vi "加标回收量程配置界面.vi"(3 "量程选择簇":T1={"氨氮推荐量程"=enum."AUTO", "总氮推荐量程"=enum."AUTO", "总磷推荐量程"=enum."AUTO", "CODMn推荐量程"=enum."H", "CODCr推荐量程"=enum."H"}, 11 "倒计时":u16) -> (2 "布尔":bool=TRUE)   [LabVIEW 2016]
uses:
  <vilib>/Utility/miscctls.llb/LVPointTypeDef.ctl
  <vilib>/Utility/config.llb/NI_LVConfig.lvlib
panel:
  in  "确认":bool
  in  "返回":bool
  in  "详情":bool
  out "CODCr 2":dbl
  out "CODMn 2":dbl
  out "总磷 2":dbl
  out "总氮 2":dbl
  out "氨氮 2":dbl
  in  "取消":bool
  out "CODCr":dbl
  out "CODMn":dbl
  out "总磷":dbl
  out "总氮":dbl
  out "氨氮":dbl
  out "CODCr下限":dbl
  out "CODCr上限":dbl
  out "CODMn下限":dbl
  out "CODMn上限":dbl
  out "总磷下限":dbl
  out "总磷上限":dbl
  out "总氮下限":dbl
  out "总氮上限":dbl
  out "氨氮下限":dbl
  out "氨氮上限":dbl
  # "加标回收量程选择"
  # "最近一组水样测试结果"
  # "加标后的理论浓度"
  # "氨氮低量程范围"
  # "~"
  # "总氮低量程范围"
  # "~"
  # "总磷低量程范围"
  # "~"
  # "~"
  # "CODMn低量程范围"
  # "~"
  # "CODCr低量程范围"
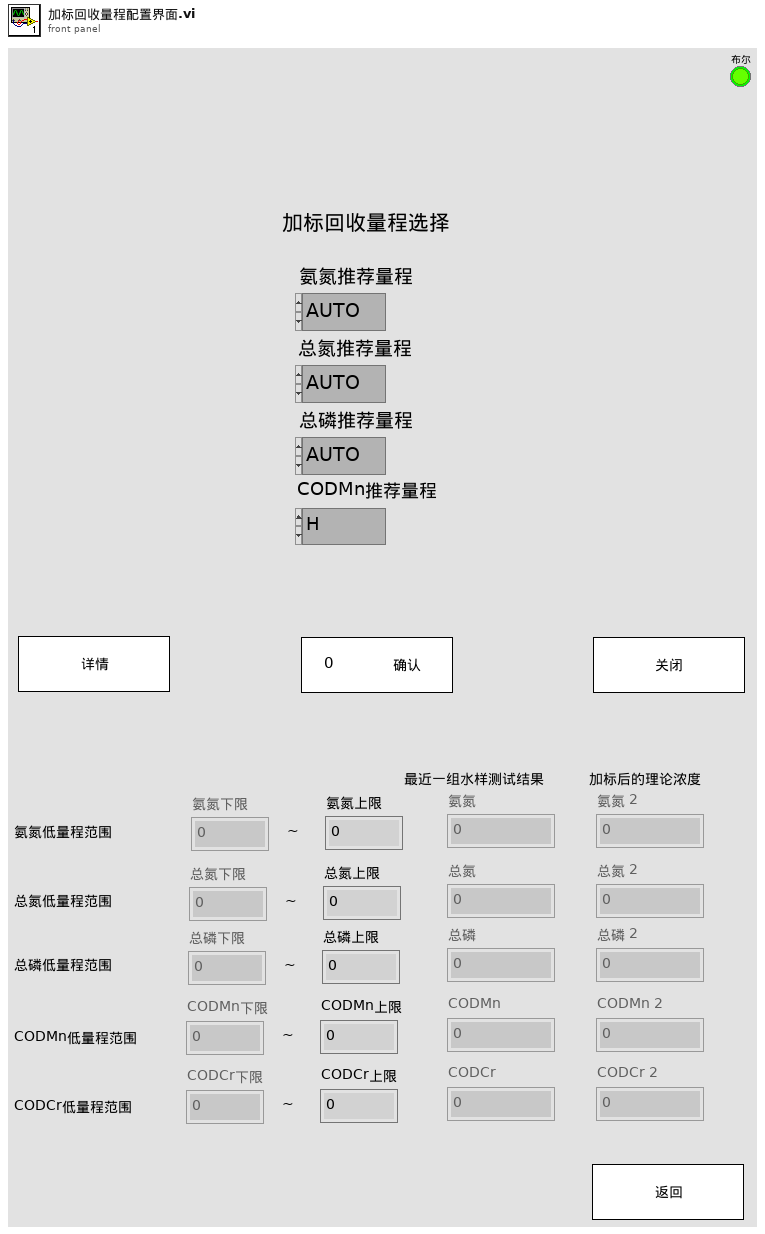
[diagram p1: front panel]
types:
  T1 = cluster{"氨氮推荐量程":enum32{"H", "L", "AUTO"}, "总氮推荐量程":enum32{"H", "L", "AUTO"}, "总磷推荐量程":enum32{"H", "L", "AUTO"}, "CODMn推荐量程":enum32{"H", "L", "AUTO"}, "CODCr推荐量程":enum32{"H", "L", "AUTO"}}
  T2 = cluster{"量程":dbl, "检出限":dbl, "加标前水样浓度":dbl, "加标后水样浓度":dbl, "加标水杯定容体积":dbl, "加标母液浓度":dbl, "加标体积":dbl, "加标回收率":dbl}
  T3 = typedef "NI_LVConfig.lvlib/Config Data RefNum.ctl" = refnum<k1>
  T4 = typedef "LVPointTypeDef.ctl" = cluster{"Horizontal":i16, "Vertical":i16}
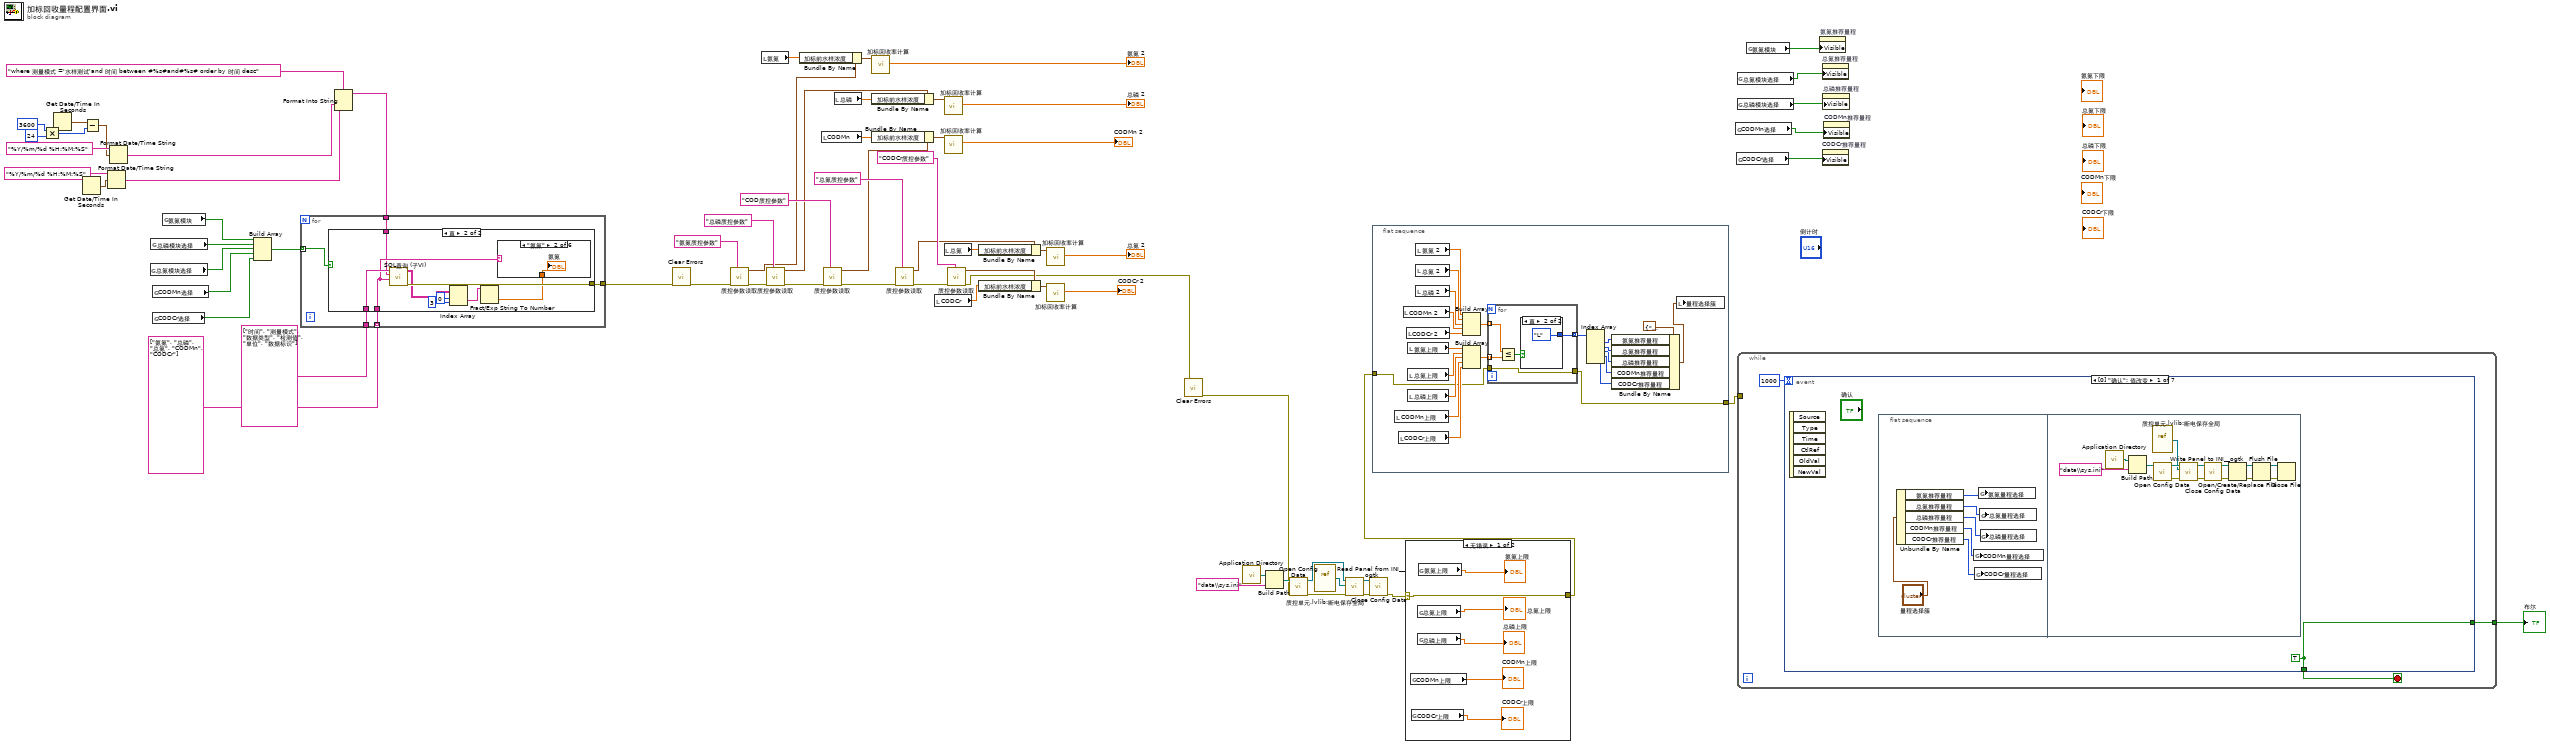
[diagram p0: block diagram]
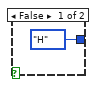
[diagram p2: hidden frame]
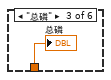
[diagram p5: hidden frame]
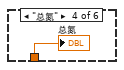
[diagram p6: hidden frame]
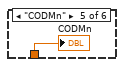
[diagram p7: hidden frame]
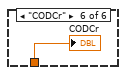
[diagram p8: hidden frame]
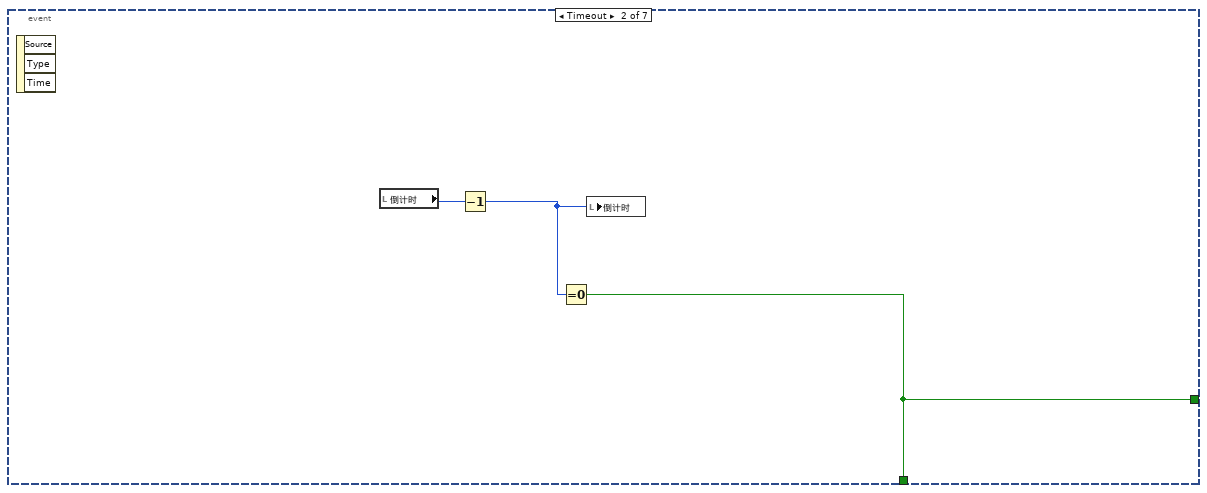
[diagram p10: hidden frame]
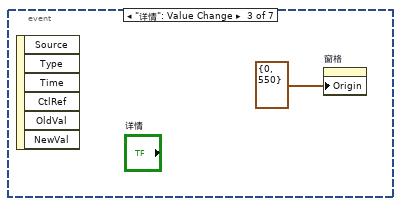
[diagram p11: hidden frame]
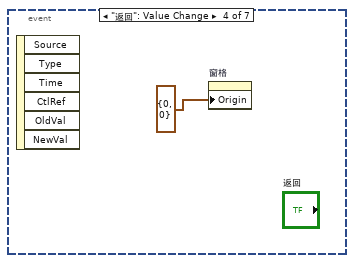
[diagram p12: hidden frame]
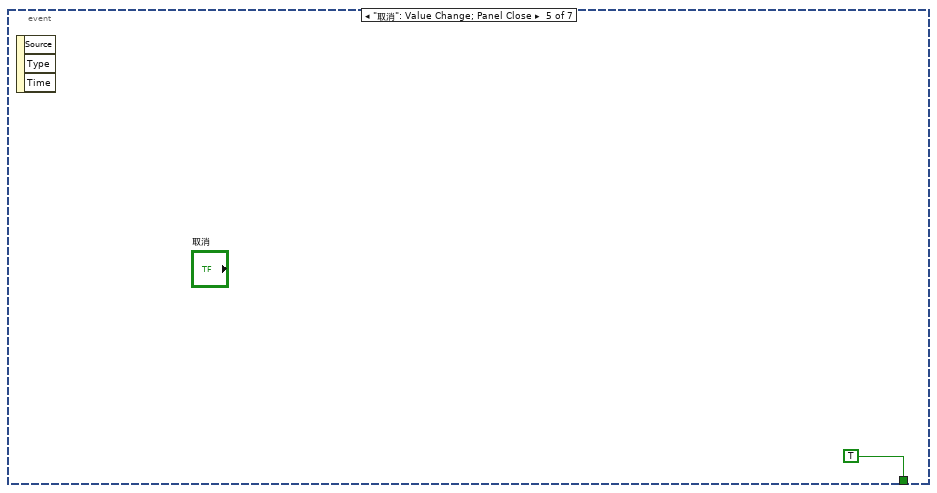
[diagram p13: hidden frame]
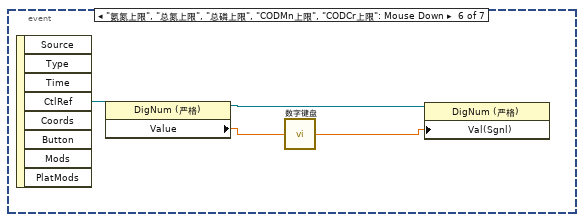
[diagram p14: hidden frame]
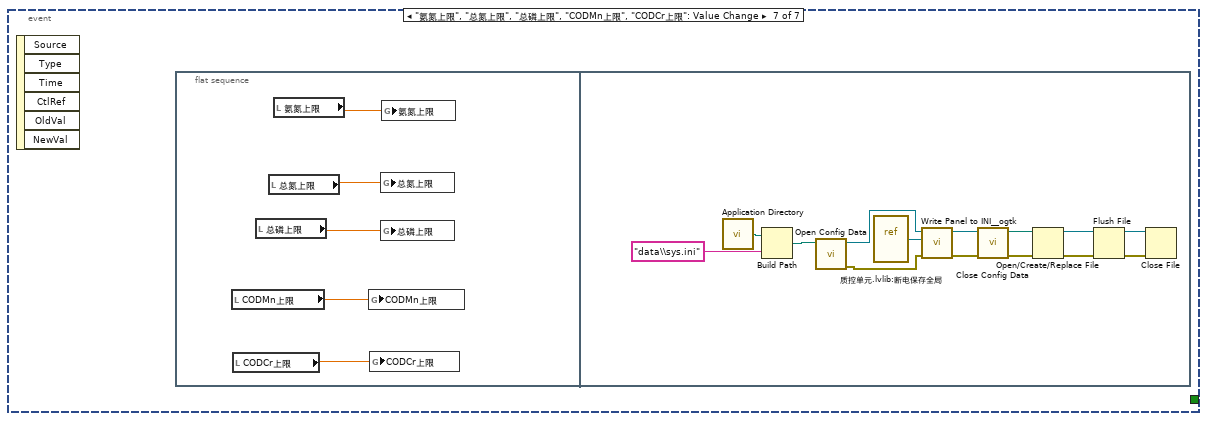
[diagram p15: hidden frame]
diagram:
  n1 = Multiply(x=3600, y=24) -> (x*y=w46:i32)
  n2 = Get Date/Time In Seconds() -> (seconds since 1Jan1904=w50:timestamp)
  n3 = Get Date/Time In Seconds() -> (seconds since 1Jan1904=w53:timestamp)
  n4 = Subtract(x=w50, y=w46) -> (x-y=w49:timestamp)
  n5 = Format Date/Time String(time format string (%c)="%Y/%m/%d %H:%M:%S" ("时间格式字符串(%c)"), seconds (now)=w53) -> (date/time string=w43:string)  [unwired: 1 in]
  n6 = Format Date/Time String(time format string (%c)="%Y/%m/%d %H:%M:%S" ("时间格式字符串(%c)"), seconds (now)=w49) -> (date/time string=w44:string)  [unwired: 1 in]
  n7 = global read "断电保存全局.vi" "总氮模块选择"() -> (w59:bool)
  n8 = global read "断电保存全局.vi" "总磷模块选择"() -> (w60:bool)
  n9 = global read "断电保存全局.vi" "CODMn选择"() -> (w58:bool)
  n10 = global read "断电保存全局.vi" "CODCr选择"() -> (w57:bool)
  n11 = global read "断电保存全局.vi" "氨氮模块"() -> (w61:bool)
  n12 = Build Array(w61, w60, w59, w58, w57) -> (w56:bool[])
  n13 = Format Into String(format string="where 测量模式 ='水样测试'and 时间 between #%s#and#%s# order by 时间 desc", w44, w43) -> (resulting string=w42:string)  [unwired: 2 in, 1 out]
  n14 = for {
    tunnel: w56 -> [w75] mode=indexing
    tunnel: string[] ["氨氮", "总磷", "总氮", "CODMn", "CODCr"] -> [w74] mode=indexing
    tunnel: string[] ["时间", "测量模式", "数据类型", "检测值", "单位", "数据标识"] ("columns") -> [w73]
    tunnel: [w72] -> w32
    tunnel: w42 -> [w71]
    n15 = case shown="真" w75 {
      tunnel: w74 -> [_ w82]
      tunnel: w73 -> [_ w84]
      tunnel: [_ w83] -> w72
      tunnel: w71 -> [_ w81]
      frame False {
      }
      frame True {
        n16 = call "SQL查询 (子VI).vi"("table输入"=w82, "condition"=w81, "columns"=w84) -> ("错误输出"=w83:errorcluster, "data"=w77:string[][])  [unwired: 7 in]
        n17 = Index Array(array=w77, index (row)=0 ("索引 (行)"), index (col)=3 ("禁用的索引 (列)")) -> (element=w80:string)
        n18 = Fract/Exp String To Number(string=w80) -> (number=w76:dbl)  [unwired: 3 in, 1 out]
        n19 = case shown="\"氨氮\"" w82 {
          tunnel: w76 -> [_ w85 w86 w87 w88 w89]
          frame "假", Default {
          }
          frame "氨氮" {
            "氨氮" <- w85
          }
          frame "总磷" {
            "总磷" <- w86
          }
          frame "总氮" {
            "总氮" <- w87
          }
          frame "CODMn" {
            "CODMn" <- w88
          }
          frame "CODCr" {
            "CODCr" <- w89
          }
        }
      }
    }
  }
  n20 = call <vilib>:"Clear Errors.vi"("error in (no error)"=w32) -> ("error out"=w31:errorcluster)  [unwired: 5 in, 1 out]
  n21 = call "质控参数读取.vi"("section"="氨氮质控参数", "error in (no error)"=w31) -> ("error out"=w39:errorcluster, "参数"=w30:T2)  [unwired: 8 in]
  n22 = local read "氨氮"() -> (w29:dbl)
  n23 = call "质控参数读取.vi"("section"="总磷质控参数", "error in (no error)"=w39) -> ("error out"=w37:errorcluster, "参数"=w24:T2)  [unwired: 8 in]
  n24 = Bundle By Name(cluster=w30, "加标前水样浓度"=w29) -> (w28:T2)
  n25 = local read "CODMn"() -> (w21:dbl)
  n26 = call "质控参数读取.vi"("section"="COD质控参数", "error in (no error)"=w37) -> ("error out"=w35:errorcluster, "参数"=w20:T2)  [unwired: 8 in]
  n27 = local read "总磷"() -> (w25:dbl)
  n28 = call "加标回收率计算.vi"("参数"=w28) -> ("加标后理论浓度"=→"氨氮 2":dbl)  [unwired: 9 in, 1 out]
  n29 = Bundle By Name(cluster=w24, "加标前水样浓度"=w25) -> (w26:T2)
  n30 = Bundle By Name(cluster=w20, "加标前水样浓度"=w21) -> (w22:T2)
  n31 = call "质控参数读取.vi"("section"="总氮质控参数", "error in (no error)"=w35) -> ("error out"=w33:errorcluster, "参数"=w16:T2)  [unwired: 8 in]
  n32 = local read "CODCr"() -> (w13:dbl)
  n33 = call "加标回收率计算.vi"("参数"=w26) -> ("加标后理论浓度"=→"总磷 2":dbl)  [unwired: 9 in, 1 out]
  n34 = call "加标回收率计算.vi"("参数"=w22) -> ("加标后理论浓度"=→"CODMn 2":dbl)  [unwired: 9 in, 1 out]
  n35 = local read "总氮"() -> (w18:dbl)
  n36 = call "质控参数读取.vi"("section"="CODCr质控参数", "error in (no error)"=w33) -> ("error out"=w10:errorcluster, "参数"=w12:T2)  [unwired: 8 in]
  n37 = Bundle By Name(cluster=w16, "加标前水样浓度"=w18) -> (w17:T2)
  n38 = Bundle By Name(cluster=w12, "加标前水样浓度"=w13) -> (w14:T2)
  n39 = call "加标回收率计算.vi"("参数"=w17) -> ("加标后理论浓度"=→"总氮 2":dbl)  [unwired: 9 in, 1 out]
  n40 = call "加标回收率计算.vi"("参数"=w14) -> ("加标后理论浓度"=→"CODCr 2":dbl)  [unwired: 9 in, 1 out]
  n41 = call <vilib>:"Clear Errors.vi"("error in (no error)"=w10) -> ("error out"=w9:errorcluster)  [unwired: 5 in, 1 out]
  n42 = call <vilib>:"Application Directory.vi"() -> ("Application Directory"=w70:path)
  n43 = Build Path(base path=w70, name or relative path="data\\sys.ini" ("名称或相对路径")) -> (appended path=w68:path)
  n44 = call <vilib>:"Open Config Data.vi"("error in (no error)"=w9, "configuration file path"=w68) -> ("error out"=w64:errorcluster, "refnum"=w67:T3)  [unwired: 7 in, 1 out]
  n45 = vi-ref "质控单元.lvlib:断电保存全局.vi"() -> (w66:refnum<vi>)
  n46 = call <userlib>:"Read Panel from INI__ogtk.vi"("error in (no error)"=w64, "VI ref"=w66, "refnum"=w67) -> ("error out"=w63:errorcluster, "refnum out"=w65:T3)  [unwired: 7 in]
  n47 = call <vilib>:"Close Config Data.vi"("error in (no error)"=w63, "refnum"=w65) -> ("error out"=w62:errorcluster)  [unwired: 8 in, 1 out]
  n48 = flat-sequence {
    tunnel: w8 -> [w98]
    tunnel: [w97] -> w7
    frame #0 {
      n49 = local read "CODMn上限"() -> (w102:dbl)
      n50 = local read "CODCr上限"() -> (w101:dbl)
      n51 = local read "CODMn 2"() -> (w107:dbl)
      n52 = local read "CODCr 2"() -> (w108:dbl)
      n53 = local read "氨氮上限"() -> (w105:dbl)
      n54 = local read "总氮上限"() -> (w104:dbl)
      n55 = local read "总磷上限"() -> (w103:dbl)
      n56 = local read "氨氮 2"() -> (w111:dbl)
      n57 = local read "总氮 2"() -> (w110:dbl)
      n58 = local read "总磷 2"() -> (w109:dbl)
      n59 = Build Array(w111, w110, w109, w107, w108) -> (w106:dbl[])
      n60 = Build Array(w105, w104, w103, w102, w101) -> (w100:dbl[])
      n61 = for {
        tunnel: w106 -> [w116] mode=indexing
        tunnel: w100 -> [w115] mode=indexing
        tunnel: [w114] -> w99 mode=indexing
        tunnel: w98 -> [w112]
        tunnel: [w112] -> w97
        n62 = Less Or Equal?(x=w116, y=w115) -> (x <= y?=w113:bool)
        n63 = case shown="真" w113 {
          tunnel: [enum32{"H", "L", "AUTO"}."H" ("氨氮推荐量程") enum32{"H", "L", "AUTO"}."L" ("氨氮推荐量程")] -> w114
          frame False {
          }
          frame True {
          }
        }
      }
      n64 = Index Array(array=w99) -> (element #1=w95:enum32{"H", "L", "AUTO"}, element #2=w94:enum32{"H", "L", "AUTO"}, element #3=w93:enum32{"H", "L", "AUTO"}, element #4=w92:enum32{"H", "L", "AUTO"}, element #5=w91:enum32{"H", "L", "AUTO"})  [unwired: 5 in]
      n65 = Bundle By Name(cluster=T1 {"氨氮推荐量程"=enum."H", "总氮推荐量程"=enum."H", "总磷推荐量程"=enum."H", "CODMn推荐量程"=enum."H", "CODCr推荐量程"=enum."H"} ("量程选择簇"), "氨氮推荐量程"=w95, "总氮推荐量程"=w94, "总磷推荐量程"=w93, "CODMn推荐量程"=w92, "CODCr推荐量程"=w91) -> (w90:T1)
      n66 = local write "量程选择簇"(w90) -> ()
    }
  }
  n67 = case shown="无错误" w62 {
    selector: w62 -> [w119 w125]
    tunnel: [w119 w125] -> w8
    frame No Error {
      n68 = global read "断电保存全局.vi" "CODMn上限"() -> (→"CODMn上限":dbl)
      n69 = global read "断电保存全局.vi" "CODCr上限"() -> (→"CODCr上限":dbl)
      n70 = global read "断电保存全局.vi" "总氮上限"() -> (→"总氮上限":dbl)
      n71 = global read "断电保存全局.vi" "总磷上限"() -> (→"总磷上限":dbl)
      n72 = global read "断电保存全局.vi" "氨氮上限"() -> (→"氨氮上限":dbl)
    }
    frame Error {
    }
  }
  n73 = global read "断电保存全局.vi" "CODMn选择"() -> (w3:bool)
  n74 = global read "断电保存全局.vi" "CODCr选择"() -> (w4:bool)
  n75 = global read "断电保存全局.vi" "总氮模块选择"() -> (w1:bool)
  n76 = global read "断电保存全局.vi" "总磷模块选择"() -> (w2:bool)
  n77 = while {
    tunnel: w7 -> [_]
    tunnel: [w127] -> w6
    stop <- w128 stop-if-true
    n78 = event shown="[0] \"确认\": 值改变" {
      selector: _ -> [_ _ _ _ _ _ _]
      dyn-events: _ -> [_ _ _ _ _ _ _]
      timeout: 1000 -> [_ _ _ _ _ _ _]
      tunnel: [w129 w151 _ _ TRUE _ _] -> w128
      tunnel: [w129 w151 _ _ _ _ _] -> w127
      event "确认": Value Change {
        w129 = TRUE
        n79 = event-data() -> ()  [unwired: 1 in, 6 out]
        n80 = flat-sequence {
          frame #0 {
            n81 = Unbundle By Name("量程选择簇") -> ("氨氮推荐量程"=w135:enum32{"H", "L", "AUTO"}, "总氮推荐量程"=w134:enum32{"H", "L", "AUTO"}, "总磷推荐量程"=w133:enum32{"H", "L", "AUTO"}, "CODMn推荐量程"=w132:enum32{"H", "L", "AUTO"}, "CODCr推荐量程"=w131:enum32{"H", "L", "AUTO"})
            n82 = global write "断电保存全局.vi" "CODMn量程选择"(w132) -> ()
            n83 = global write "断电保存全局.vi" "CODCr量程选择"(w131) -> ()
            n84 = global write "断电保存全局.vi" "氨氮量程选择"(w135) -> ()
            n85 = global write "断电保存全局.vi" "总氮量程选择"(w134) -> ()
            n86 = global write "断电保存全局.vi" "总磷量程选择"(w133) -> ()
          }
          frame #1 {
            n87 = call <vilib>:"Application Directory.vi"() -> ("Application Directory"=w149:path)
            n88 = Build Path(base path=w149, name or relative path="data\\sys.ini" ("名称或相对路径")) -> (appended path=w147:path)
            n89 = vi-ref "质控单元.lvlib:断电保存全局.vi"() -> (w145:refnum<vi>)
            n90 = call <vilib>:"Open Config Data.vi"("configuration file path"=w147) -> ("error out"=w143:errorcluster, "refnum"=w146:T3)  [unwired: 8 in, 1 out]
            n91 = call <userlib>:"Write Panel to INI__ogtk.vi"("error in (no error)"=w143, "VI ref"=w145, "refnum"=w146) -> ("error out"=w142:errorcluster, "refnum out"=w144:T3)  [unwired: 7 in]
            n92 = call <vilib>:"Close Config Data.vi"("error in (no error)"=w142, "refnum"=w144) -> ("error out"=w137:errorcluster, "file path"=w136:path)  [unwired: 8 in]
            n93 = Open/Create/Replace File(file path (use dialog)=w136, error in=w137) -> (refnum out=w140:refnum<file>, error out=w141:errorcluster)  [unwired: 4 in, 1 out]
            n94 = Flush File(refnum=w140, error in=w141) -> (refnum out=w139:refnum<file>, error out=w138:errorcluster)
            n95 = Close File(refnum=w139, error in=w138) -> ()  [unwired: 2 out]
          }
        }
      }
      event Timeout {
        n96 = event-data() -> ()  [unwired: 1 in, 3 out]
        n97 = local read "倒计时"() -> (w152:u16)
        n98 = Decrement(x=w152) -> (x-1=w150:u16)
        n99 = Equal To 0?(x=w150) -> (x = 0?=w151:bool)
        n100 = local write "倒计时"(w150) -> ()
      }
      event "详情": Value Change {
        n101 = event-data() -> ()  [unwired: 1 in, 6 out]
        n102 = property on="窗格" class="Pane"("Origin"=T4 {"Horizontal"=0, "Vertical"=550} ("原点")) -> ()  [unwired: 2 in, 2 out]
      }
      event "返回": Value Change {
        n103 = event-data() -> ()  [unwired: 1 in, 6 out]
        n104 = property on="窗格" class="Pane"("Origin"=T4 {"Horizontal"=0, "Vertical"=0} ("原点")) -> ()  [unwired: 2 in, 2 out]
      }
      event "取消": Value Change; Panel Close {
        n105 = event-data() -> ()  [unwired: 1 in, 3 out]
      }
      event "氨氮上限", "总氮上限", "总磷上限", "CODMn上限", "CODCr上限": Mouse Down {
        n106 = event-data() -> ("CtlRef"=w159:refnum<vi>)  [unwired: 1 in, 7 out]
        n107 = property class="DigNum (严格)"(reference=w159) -> (reference out=w157:refnum<vi>, "Value"=w158:dbl)  [unwired: 1 in, 1 out]
        n108 = call "数字键盘.vi"("OldNumber"=w158) -> ("NewNumber"=w156:sgl)
        n109 = property class="DigNum (严格)"(reference=w157, "Val(Sgnl)"=w156) -> ()  [unwired: 1 in, 2 out]
      }
      event "氨氮上限", "总氮上限", "总磷上限", "CODMn上限", "CODCr上限": Value Change {
        n110 = event-data() -> ()  [unwired: 1 in, 6 out]
        n111 = flat-sequence {
          frame #0 {
            n112 = local read "CODMn上限"() -> (w161:dbl)
            n113 = local read "CODCr上限"() -> (w160:dbl)
            n114 = local read "总磷上限"() -> (w162:dbl)
            n115 = local read "总氮上限"() -> (w163:dbl)
            n116 = local read "氨氮上限"() -> (w164:dbl)
            n117 = global write "断电保存全局.vi" "CODMn上限"(w161) -> ()
            n118 = global write "断电保存全局.vi" "CODCr上限"(w160) -> ()
            n119 = global write "断电保存全局.vi" "总氮上限"(w163) -> ()
            n120 = global write "断电保存全局.vi" "总磷上限"(w162) -> ()
            n121 = global write "断电保存全局.vi" "氨氮上限"(w164) -> ()
          }
          frame #1 {
            n122 = call <vilib>:"Application Directory.vi"() -> ("Application Directory"=w178:path)
            n123 = Build Path(base path=w178, name or relative path="data\\sys.ini" ("名称或相对路径")) -> (appended path=w176:path)
            n124 = call <vilib>:"Open Config Data.vi"("configuration file path"=w176) -> ("error out"=w172:errorcluster, "refnum"=w175:T3)  [unwired: 8 in, 1 out]
            n125 = vi-ref "质控单元.lvlib:断电保存全局.vi"() -> (w174:refnum<vi>)
            n126 = call <userlib>:"Write Panel to INI__ogtk.vi"("error in (no error)"=w172, "VI ref"=w174, "refnum"=w175) -> ("error out"=w171:errorcluster, "refnum out"=w173:T3)  [unwired: 7 in]
            n127 = call <vilib>:"Close Config Data.vi"("error in (no error)"=w171, "refnum"=w173) -> ("error out"=w166:errorcluster, "file path"=w165:path)  [unwired: 8 in]
            n128 = Open/Create/Replace File(file path (use dialog)=w165, error in=w166) -> (refnum out=w169:refnum<file>, error out=w170:errorcluster)  [unwired: 4 in, 1 out]
            n129 = Flush File(refnum=w169, error in=w170) -> (refnum out=w168:refnum<file>, error out=w167:errorcluster)
            n130 = Close File(refnum=w168, error in=w167) -> ()  [unwired: 2 out]
          }
        }
      }
    }
  }
  "布尔" <- w6
  n131 = global read "断电保存全局.vi" "氨氮模块"() -> (w5:bool)
  n132 = property on="氨氮推荐量程" class="Enum (严格)"("Visible"=w5) -> ()  [unwired: 2 in, 2 out]
  n133 = property on="总氮推荐量程" class="Enum (严格)"("Visible"=w1) -> ()  [unwired: 2 in, 2 out]
  n134 = property on="CODCr推荐量程" class="Enum (严格)"("Visible"=w4) -> ()  [unwired: 2 in, 2 out]
  n135 = property on="总磷推荐量程" class="Enum (严格)"("Visible"=w2) -> ()  [unwired: 2 in, 2 out]
  n136 = property on="CODMn推荐量程" class="Enum (严格)"("Visible"=w3) -> ()  [unwired: 2 in, 2 out]
